vi "Display Data List.vi"(6 "Peak List":T1[](array[typedef]), 9 "Data Type":enum16{"TIC", "Spectrum", "Peak"}(ring)) -> ()   [LabVIEW 2012]
uses:
  Type/_Peak Property.ctl
  <vilib>/Utility/miscctls.llb/LVRectTypeDef.ctl
  Type/_Data Operation.ctl
  <vilib>/Utility/file.llb/Write To Spreadsheet File (DBL).vi
panel:
  in  "Export":bool
  out "Data":i32(listbox) caption="Peak Data"
  out "Total # of Rows":i32=4 min=2 max=100
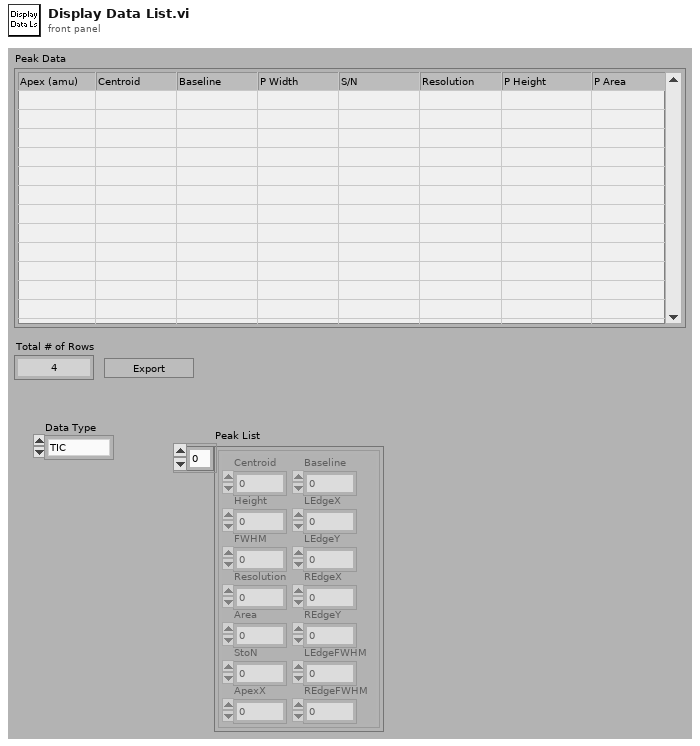
[diagram p1: front panel]
types:
  T1 = typedef "_Peak Property.ctl" = cluster{"Centroid":dbl, "Height":dbl, "FWHM":dbl, "Resolution":dbl, "Area":dbl, "StoN":dbl, "ApexX":dbl, "Baseline":dbl, "LEdgeX":dbl, "LEdgeY":dbl, "REdgeX":dbl, "REdgeY":dbl, "LEdgeFWHM":dbl, "REdgeFWHM":dbl}
  T2 = typedef "_Data Operation.ctl" = enum8{"Initialize", "Get Data", "Set Data", "Close"}
  T3 = typedef "LVRectTypeDef.ctl" = cluster{"Left":i16, "Top":i16, "Right":i16, "Bottom":i16}
  T4 = typedef "_Current Data.ctl" = cluster{"Scan#":i32, "Run Time (mS)":i32, "TIC X":dbl[], "TIC Y":dbl[][], "MassRange":cluster{"X Title":string, "X":dbl[], "Y":i32[]}[], "Fixed Mass (amu)":dbl, "Method":T5}
  T5 = typedef "_XML Expt.ctl" = cluster{"StartT(mS)":i32, "#Cycles":i32, "PauseT(uS)":i32, "ScanType":i32, "Polarity":u8, "FixedMass":dbl, "DelayT(mS)":i32, "Active Ch":T6[], "Mass Range":T7[]}
  T6 = typedef "_XML Lens.ctl" = cluster{"Value":dbl, "ChID":u8}
  T7 = typedef "_Mass Range Property.ctl" = cluster{"Start":dbl, "Stop":dbl, "Step Size":dbl, "Steps":i32, "Dwell":dbl, "Parameters":T8[], "Res":T9}
  T8 = typedef "_Mass Range Parameters.ctl" = cluster{"Name":string, "Ch#":u8, "StartV":dbl, "StopV":dbl, "StepV":dbl, "Index":u8}
  T9 = typedef "_RT Res Type.ctl" = u16
  T10 = cluster{"X Title":string, "X":dbl[], "Y":i32[]}[]
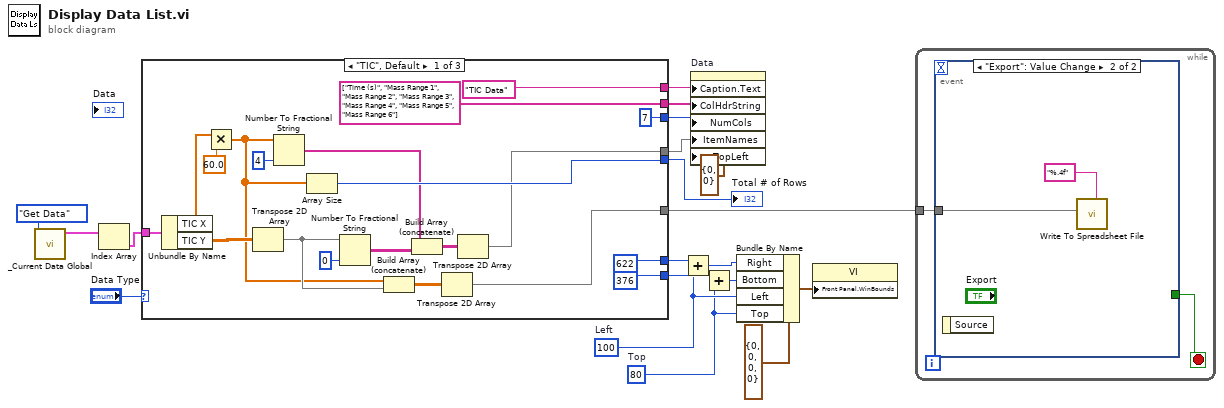
[diagram p0: block diagram]
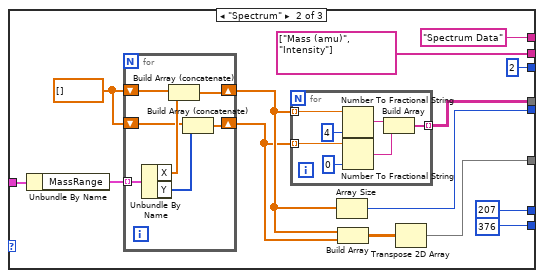
[diagram p2: hidden frame]
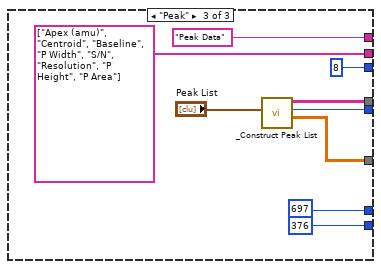
[diagram p3: hidden frame]
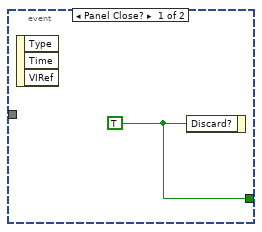
[diagram p4: hidden frame]
diagram:
  w6 = i16 80  # Top
  w7 = i16 100  # Left
  n1 = call "_Current Data Global.vi"("Operation"=_Data_Operation."Get Data") -> ("CurrentData"=w2:T4[])  [unwired: 3 in, 3 out]
  n2 = Index Array(array=w2) -> (element=w1:T4)  [unwired: 1 in]
  n3 = case shown="\"TIC\", Default" "Data Type" {
    tunnel: [string[] ["Time (s)", "Mass Range 1", "Mass Range 2", "Mass Range 3", "Mass Range 4", "Mass Range 5", "Mass Range 6"] string[] ["Mass (amu)", "Intensity"] string[] ["Apex (amu)", "Centroid", "Baseline", "P Width", "S/N", "Resolution", "P Height", "P Area"]] -> w17
    tunnel: ["TIC Data" "Spectrum Data" "Peak Data"] -> w18
    tunnel: [u32 7 u32 2 u32 8] -> w16
    tunnel: [i16 622 ("right") i16 207 ("right") i16 697 ("right")] -> w15
    tunnel: [i16 376 ("right") i16 376 ("right") i16 376 ("right")] -> w13
    tunnel: [w23 w47 w70] -> w10
    tunnel: [w34 w46 w69] -> w5
    tunnel: [w32 w45 w68] -> w9
    tunnel: w1 -> [w30 w44 _]
    frame "TIC", Default {
      n4 = Unbundle By Name(w30) -> ("TIC X"=w22:dbl[], "TIC Y"=w29:dbl[][])
      n5 = Multiply(x=w22, y=60.0 ("precision (6)")) -> (x*y=w20:dbl[])
      n6 = Transpose 2D Array(2D array=w29) -> (transposed array=w27:dbl[][])
      n7 = Number To Fractional String(number=w20, precision (6)=i16 4) -> (F-format string=w25:string[])  [unwired: 2 out]
      n8 = Array Size(array=w20) -> (size(s)=w34:i32)
      n9 = Number To Fractional String(number=w27, precision (6)=i16 0) -> (F-format string=w26:string[][])  [unwired: 2 out]
      n10 = Build Array (concatenate)(w20, w27) -> (w33:dbl[][])
      n11 = Build Array (concatenate)(w25, w26) -> (w24:string[][])
      n12 = Transpose 2D Array(2D array=w33) -> (transposed array=w32:dbl[][])
      n13 = Transpose 2D Array(2D array=w24) -> (transposed array=w23:string[][])
    }
    frame "Spectrum" {
      w42 = dbl[] []
      n14 = Unbundle By Name(w44) -> ("MassRange"=w43:T10)
      n15 = for {
        tunnel: w43 -> [w60] mode=indexing
        shift-right: [w55] -> w41
        shift-left: w42 -> [w54]
        shift-right: [w57] -> w40
        shift-left: w42 -> [w56]
        n16 = Unbundle By Name(w60) -> ("X"=w59:dbl[], "Y"=w58:i32[])
        n17 = Build Array (concatenate)(w54, w59) -> (w55:dbl[])
        n18 = Build Array (concatenate)(w56, w58) -> (w57:dbl[])
      }
      n19 = for {
        tunnel: w41 -> [w67] mode=indexing
        tunnel: w40 -> [w66] mode=indexing
        tunnel: [w61] -> w47 mode=indexing
        n20 = Number To Fractional String(number=w67, precision (6)=i16 4) -> (F-format string=w63:string)  [unwired: 2 out]
        n21 = Number To Fractional String(number=w66, precision (6)=i16 0) -> (F-format string=w62:string)  [unwired: 2 out]
        n22 = Build Array(w63, w62) -> (w61:string[])
      }
      n23 = Array Size(array=w41) -> (size(s)=w46:i32)
      n24 = Build Array(w41, w40) -> (w48:dbl[][])
      n25 = Transpose 2D Array(2D array=w48) -> (transposed array=w45:dbl[][])
    }
    frame "Peak" {
      n26 = call "_Construct Peak List.vi"("Peak List"="Peak List") -> ("Array"=w68:dbl[][], "# of Peaks"=w69:i32, "Table"=w70:string[][])  [unwired: 2 in, 2 out]
    }
  }
  "Total # of Rows" <- w5
  n27 = Add(x=w15, y=w7) -> (x+y=w14:i16)
  n28 = property on="Data" class="MCListbox (strict)"("Caption.Text"=w18, "ColHdrString"=w17, "NumCols"=w16, "ItemNames"=w10, "TopLeft"=cluster{"Row":u32, "Column":u32} {"Row"=0, "Column"=0} ("Top Left Visible Cell")) -> ()  [unwired: 2 in, 2 out]
  n29 = Add(x=w13, y=w6) -> (x+y=w12:i16)
  n30 = Bundle By Name(cluster=T3 {"Left"=0, "Top"=0, "Right"=0, "Bottom"=0} ("output cluster"), "Right"=w14, "Bottom"=w12, "Left"=w7, "Top"=w6) -> (w11:T3)
  n31 = property class="VI"("Front Panel.WinBounds"=w11) -> ()  [unwired: 2 in, 2 out]
  n32 = while {
    tunnel: w9 -> [w77]
    stop <- w78 stop-if-true
    n33 = event shown="[1] \"Export\": Value Change" {
      selector: _ -> [_ _]
      dyn-events: _ -> [_ _]
      timeout: _ -> [_ _]
      tunnel: [w79 _] -> w78
      tunnel: w77 -> [_ w81]
      event Panel Close? {
        w79 = TRUE ("Discard?")
        n34 = event-data() -> ()  [unwired: 4 out]
        n35 = event-data("Discard?"=w79) -> ()  [unwired: 1 in, 1 out]
      }
      event "Export": Value Change {
        n36 = event-data() -> ()  [unwired: 2 out]
        n37 = call-poly <vilib>:"Write To Spreadsheet File.vi"("format (%.3f)"="%.4f", "2D data"=w81) -> ()  [unwired: 4 in, 3 out]
      }
    }
  }
